vi "FPGA new main.vi"() -> ()   [LabVIEW 2020]
uses:
  <vilib>/Platform/TimedLoop/XDataNode/timing_clust.ctl
  <vilib>/Platform/TimedLoop/XDataNode/nitl_modes.ctl
  <vilib>/Platform/TimedLoop/XDataNode/wakeup.ctl
  <vilib>/rvi/Emulation/niFpgaSctlEmulationGetInTimedLoop.vi
  <vilib>/rvi/Emulation/niFpgaEmulationReportErrorSimple.vi
  <vilib>/rvi/Emulation/niFpgaGetClockAttributes.vi
  <vilib>/rvi/Emulation/niFpgaCriticalErrorInLSC.vi
  <vilib>/rvi/eio/common/nirviEmuTemplateMethod_errors.vi
  <vilib>/rvi/interface/RandomDataEmulation/niFpgaRandomDataHandleErrors.vi
  <vilib>/Platform/TimedLoop/XDataNode/XDataNode.xnode
  <vilib>/eio/EIONode/EIONode.xnode
  <vilib>/rvi/DataTransferAndStorage/Container/XNode/niFpgaContainer.xnode
  <vilib>/rvi/interface/RandomDataEmulation/nirviRandomDataFpgaReadWriteTemplate.vi
  <vilib>/Platform/TimedLoop/XDataNode/XDNodeRunTimeDep.lvlib
panel:
  out "Timed Out? 5":bool
  out "Timed Out? 4":bool
  out "Timed Out? 3":bool
  out "Timed Out? 2":bool
  out "Init Done":bool
  in  "Start Acquisition":bool
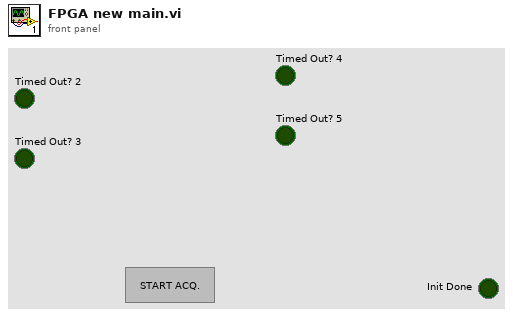
[diagram p1: front panel]
types:
  T1 = typedef "XDNodeRunTimeDep.lvlib/timing_clust.ctl" = cluster{"Expected End [f-1]":u64, "Actual End [f-1]":u64, "Finished Late? [f-1]":bool, "Expected End [i-1]":u64, "Actual End [i-1]":u64, "Finished Late? [i-1]":bool, "Expected Start [i]":u64, "Actual Start [i]":u64, "Expected Start [f]":u64, "Actual Start [f]":u64, "Source Name":string, "Structure Name":string, "Period":i64, "Deadline":i64, "Offset":i64, "Start":i64, "Priority":i32, "Timeout":i32, "Mode":T2, "Wakeup Reason":T3, "Error":errorcluster, "Source Type":string, "Secondary Source Type":string, "Global End Time":u64, "Global Start Time":u64, "Frame Duration":u64, "Iteration Duration":u64, "Assigned CPU":i32, "I/O Scan Engine Mode":u32}
  T2 = typedef "XDNodeRunTimeDep.lvlib/nitl_modes.ctl" = enum32{"No Change", "Process missed periods, maintain original phase", "Discard missed periods, maintain original phase", "Process missed periods, ignore original phase", "Discard missed periods, ignore original phase"}
  T3 = typedef "XDNodeRunTimeDep.lvlib/wakeup.ctl" = enum32{"Normal", "Aborted", "Asynchronous wakeup", "Timing source error", "Timed loop error", "Timeout"}
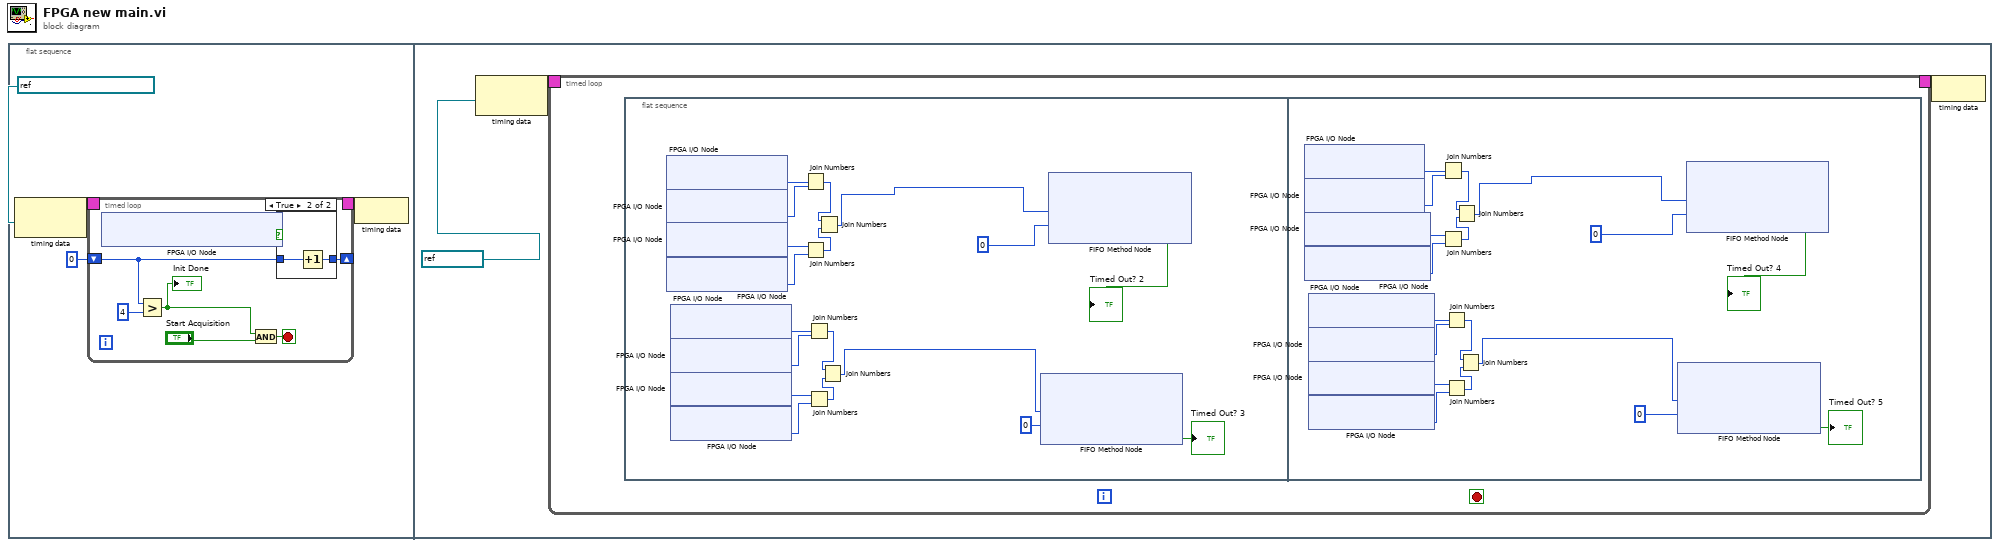
[diagram p0: block diagram]
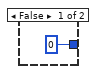
[diagram p2: hidden frame]
diagram:
  n1 = flat-sequence {
    frame #0 {
      n2 = node-c288(refnum<k21> "40 MHz Onboard Clock" ("Source Name")) -> (w4:T1)
      n3 = timed-loop {
        shift-right: [w10] -> _
        shift-left: u16 0 -> [w9]
        timing: w4 -> [_]
        timing-out: [_] -> w3
        stop <- w7 stop-if-true
        n4 = xnode "FPGA I/O Node"() -> ("IO Module\\Initialization Done"=w11:bool)  [unwired: 1 in, 1 out]
        n5 = Greater?(x=w9, y=u16 4) -> (0:w5:bool)
        "Init Done" <- w5
        n6 = And(x=w5, y="Start Acquisition") -> (x .and. y?=w7:bool)
        n7 = case shown="True" w11 {
          tunnel: [u16 0 w14] -> w10
          tunnel: w9 -> [_ w13]
          frame False {
          }
          frame True {
            n8 = Increment(x=w13) -> (x+1=w14:u16)
          }
        }
      }
      n9 = node-c288(w3) -> ()
    }
    frame #1 {
      n10 = node-c288(refnum<k21> "2.5MHz" ("Source Name")) -> (w23:T1)
      n11 = timed-loop {
        timing: w23 -> [_]
        timing-out: [_] -> w22
        stop <- _ stop-if-true
        n12 = flat-sequence {
          frame #0 {
            n13 = xnode "FPGA I/O Node"() -> ("IO Module\\AI A0"=w33:i16)  [unwired: 1 in, 1 out]
            n14 = xnode "FPGA I/O Node"() -> ("IO Module\\AI A1"=w34:i16)  [unwired: 1 in, 1 out]
            n15 = xnode "FPGA I/O Node"() -> ("IO Module\\AI A2"=w35:i16)  [unwired: 1 in, 1 out]
            n16 = xnode "FPGA I/O Node"() -> ("IO Module\\AI A3"=w30:i16)  [unwired: 1 in, 1 out]
            n17 = xnode "FPGA I/O Node"() -> ("IO Module\\AI A4"=w27:i16)  [unwired: 1 in, 1 out]
            n18 = xnode "FPGA I/O Node"() -> ("IO Module\\AI A5"=w28:i16)  [unwired: 1 in, 1 out]
            n19 = xnode "FPGA I/O Node"() -> ("IO Module\\AI A6"=w29:i16)  [unwired: 1 in, 1 out]
            n20 = xnode "FPGA I/O Node"() -> ("IO Module\\AI A7"=w24:i16)  [unwired: 1 in, 1 out]
            n21 = Join Numbers(hi=w33, lo=w34) -> ((hi.lo)=w32:u32)
            n22 = Join Numbers(hi=w35, lo=w30) -> ((hi.lo)=w31:u32)
            n23 = Join Numbers(hi=w27, lo=w28) -> ((hi.lo)=w26:u32)
            n24 = Join Numbers(hi=w29, lo=w24) -> ((hi.lo)=w25:u32)
            n25 = Join Numbers(hi=w32, lo=w31) -> ((hi.lo)=w41:u64)
            n26 = Join Numbers(hi=w26, lo=w25) -> ((hi.lo)=w38:u64)
            n27 = xnode ("FIFO Method Node")("Element"=w38, "Timeout"=0) -> ("Timed Out?"=→"Timed Out? 3":bool)  [unwired: 1 in, 1 out]
            n28 = xnode ("FIFO Method Node")("Element"=w41, "Timeout"=0) -> ("Timed Out?"=→"Timed Out? 2":bool)  [unwired: 1 in, 1 out]
          }
          frame #1 {
            n29 = xnode "FPGA I/O Node"() -> ("IO Module\\AI B8"=w51:i16)  [unwired: 1 in, 1 out]
            n30 = xnode "FPGA I/O Node"() -> ("IO Module\\AI B9"=w52:i16)  [unwired: 1 in, 1 out]
            n31 = xnode "FPGA I/O Node"() -> ("IO Module\\AI B10"=w53:i16)  [unwired: 1 in, 1 out]
            n32 = xnode "FPGA I/O Node"() -> ("IO Module\\AI B11"=w48:i16)  [unwired: 1 in, 1 out]
            n33 = xnode "FPGA I/O Node"() -> ("IO Module\\AI B12"=w45:i16)  [unwired: 1 in, 1 out]
            n34 = xnode "FPGA I/O Node"() -> ("IO Module\\AI B13"=w46:i16)  [unwired: 1 in, 1 out]
            n35 = xnode "FPGA I/O Node"() -> ("IO Module\\AI B14"=w47:i16)  [unwired: 1 in, 1 out]
            n36 = xnode "FPGA I/O Node"() -> ("IO Module\\AI B15"=w42:i16)  [unwired: 1 in, 1 out]
            n37 = Join Numbers(hi=w51, lo=w52) -> ((hi.lo)=w50:u32)
            n38 = Join Numbers(hi=w53, lo=w48) -> ((hi.lo)=w49:u32)
            n39 = Join Numbers(hi=w45, lo=w46) -> ((hi.lo)=w44:u32)
            n40 = Join Numbers(hi=w47, lo=w42) -> ((hi.lo)=w43:u32)
            n41 = Join Numbers(hi=w50, lo=w49) -> ((hi.lo)=w59:u64)
            n42 = Join Numbers(hi=w44, lo=w43) -> ((hi.lo)=w56:u64)
            n43 = xnode ("FIFO Method Node")("Element"=w56, "Timeout"=0) -> ("Timed Out?"=→"Timed Out? 5":bool)  [unwired: 1 in, 1 out]
            n44 = xnode ("FIFO Method Node")("Element"=w59, "Timeout"=0) -> ("Timed Out?"=→"Timed Out? 4":bool)  [unwired: 1 in, 1 out]
          }
        }
      }
      n45 = node-c288(w22) -> ()
    }
  }
